vi "Check_EnFlo_Tunnel_Cond.vi"(2 "Averaging time (mins)":dbl=5.0, 3 "Traverse line":T1 {"Carrier_2 Q (l/min)" format="%#.2f"; "Row Duration (mins)" format="%#.1f"; "Row No" min=0; "Trace Gas Concentration (%)" min=0.0 format="%#_4f"; "Carrier_1 Q (l/min)" format="%#.4f"; "Start X" format="%#.2f"; "Start Y" format="%#.2f"; "Start Z" format="%#.2f"; "End X" format="%#.2f"; "End Y" format="%#.2f"; "End Z" format="%#.2f"; "Tunnel Speed" format="%#.2f"; "Averaging time (mins)" min=0.0 format="%#.2f"}) -> (0 "Status Cluster":T4, 1 "Heaters On?":bool)   [LabVIEW 2021]
uses:
  Anemometry/Anemometry Sub Vis/Gen Trav/Status_Cluster.ctl
  Anemometry/Anemometry Sub Vis/Gen Trav/Multi_Run_Status.ctl
  Anemometry/Anemometry Sub Vis/Gen Trav/Traverse_cluster.ctl
  Anemometry/Anemometry Sub Vis/Gen Trav/Spacing.ctl
  Anemometry/Anemometry Sub Vis/Controls/Multi_run_mode.ctl
  Anemometry/Anemometry Sub Vis/Controls/In_Range.ctl
  Anemometry/Anemometry Sub Vis/Controls/User_Specific_mode.ctl
  Anemometry/Anemometry Sub Vis/Globals/Meas_global.vi
  Anemometry/Anemometry Sub Vis/Globals/EnFlo_Tunnel_Global.vi
  Anemometry/Anemometry Sub Vis/Globals/Trav_pos_global.vi
panel:
  # "X           Y          Z"
  # "Start"
  # "End"
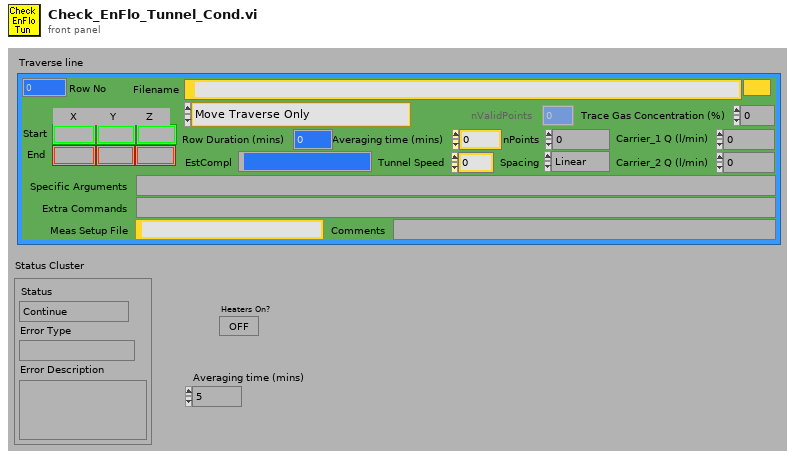
[diagram p1: front panel]
types:
  T1 = typedef "Traverse_cluster.ctl" = cluster{"Start X":sgl, "Start Y":sgl, "Start Z":sgl, "End X":sgl, "End Y":sgl, "End Z":sgl, "nPoints":i32, "Spacing":T2, "Filename":path, "Tunnel Speed":dbl, "Averaging time (mins)":dbl, "Extra Commands":string, "Carrier_1 Q (l/min)":dbl, "Carrier_2 Q (l/min)":dbl, "Trace Gas Concentration (%)":dbl, "Specific Arguments":string, "Comments":string, "Row No":i32, "Row Type Selector":T3, "EstCompl":string, "Row Duration (mins)":dbl, "nValidPoints":i32, "Meas Setup File":string}
  T2 = typedef "Spacing.ctl" = enum16{"Linear", "Log", "Gauss", "Specified", "N/A"}
  T3 = typedef "Multi_run_mode.ctl" = enum16{"Move Traverse Only", "Set Tunnel Speed Only", "Set Source Only", "Set Measurement Conditions", "Single Measurement", "Vertical Profile", "Lateral Profile", "Longitudinal Profile", "Multi-Axis Profile", "Explore Volume", "Auto Calibrate", "Meas Fast FID Bkgnd", "Check Beam Power", "Scanning Valve Measurement", "Run VI Named:", "Set ADAM Ch", "Wait (minutes)", "Send Message", "Synchronize With:", "Fall Back to this Row", "Turn Off Row Repeating", "Traverse 3D Volume", "Blank Row", "Jump to Fall Back Row"}
  T4 = typedef "Status_Cluster.ctl" = cluster{"Status":T5, "Error Type":string, "Error Description":string}
  T5 = typedef "Multi_Run_Status.ctl" = enum16{"Continue", "Continue with Error", "Jump to Next Point", "Jump to Next Row", "Jump To Fall Back", "Terminate Run"}
  T6 = typedef "In_Range.ctl" = enum16{"%", "±", "% & ±"}
  T7 = typedef "User_Specific_mode.ctl" = enum16{"Check VI only", "Run VI"}
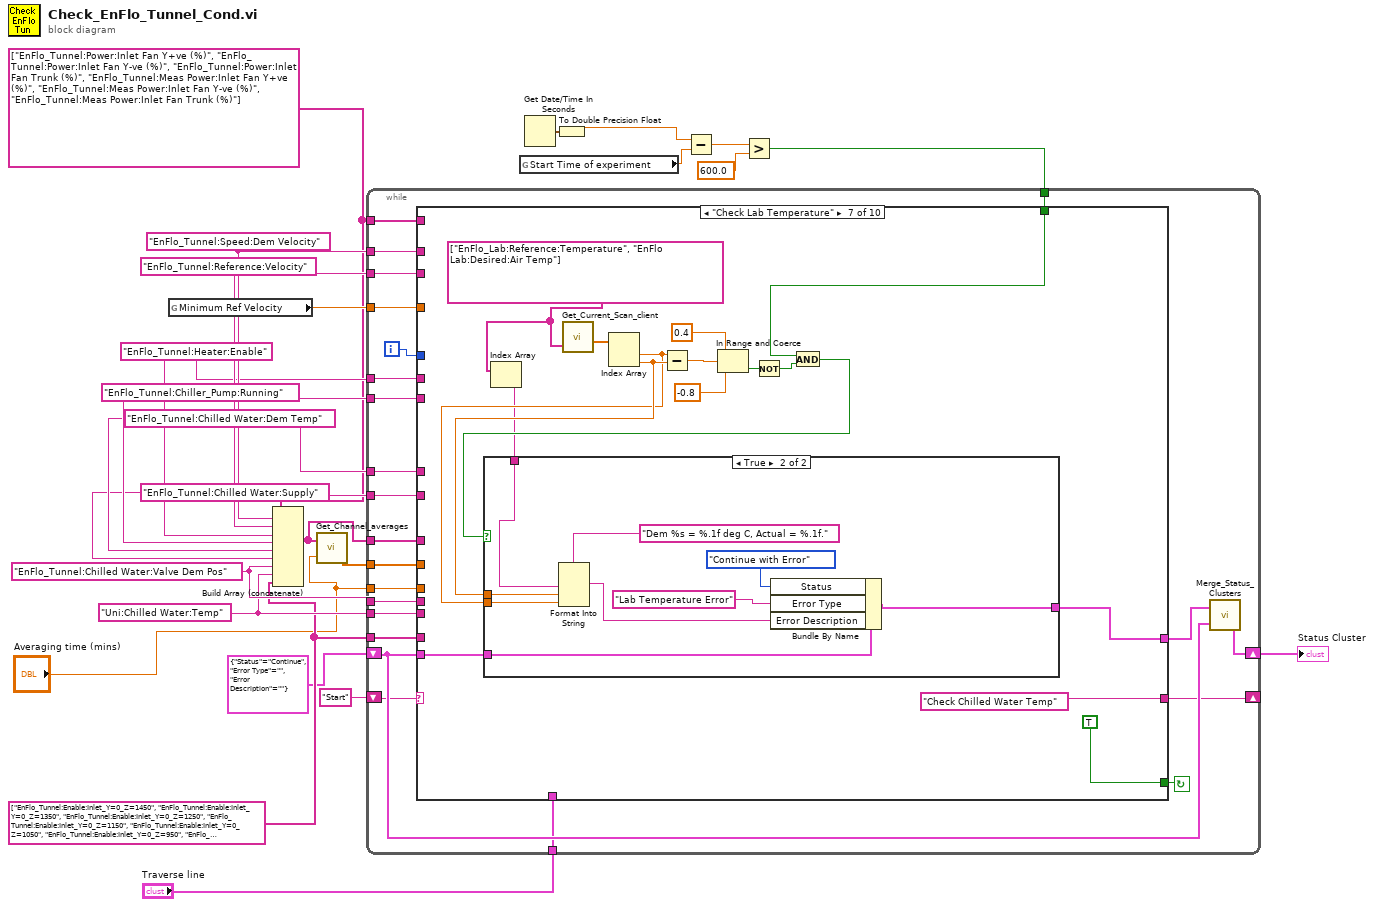
[diagram p0: block diagram]
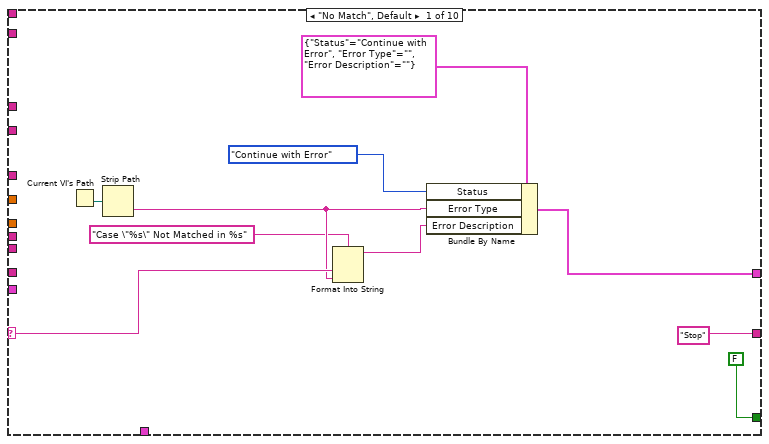
[diagram p2: hidden frame]
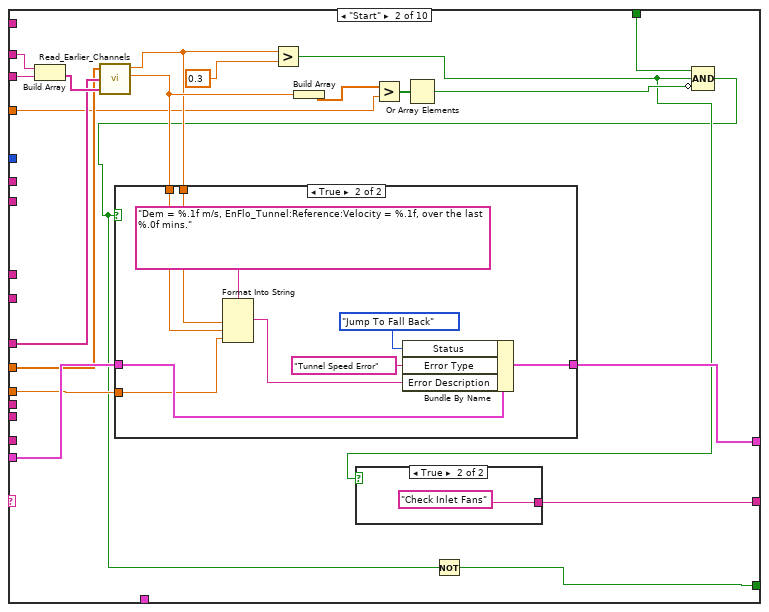
[diagram p3: hidden frame]
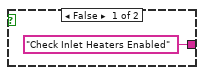
[diagram p4: hidden frame]
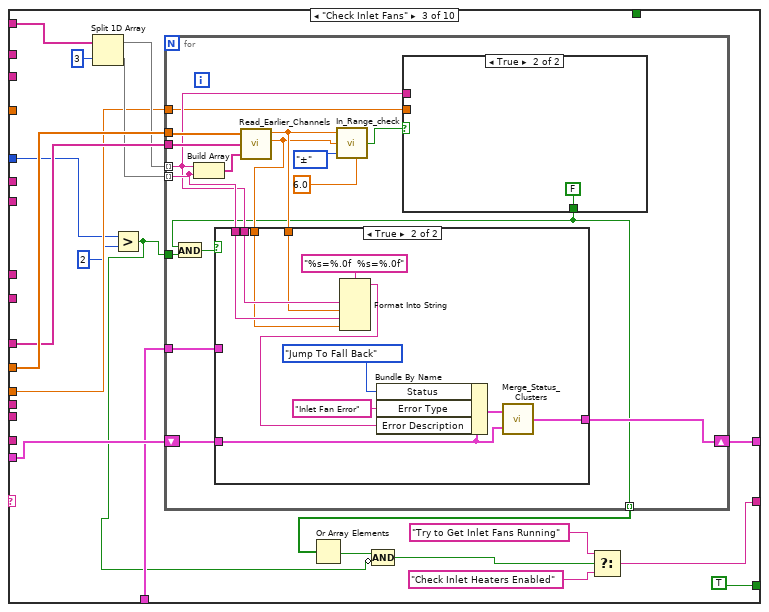
[diagram p6: hidden frame]
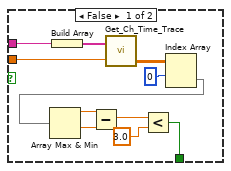
[diagram p7: hidden frame]
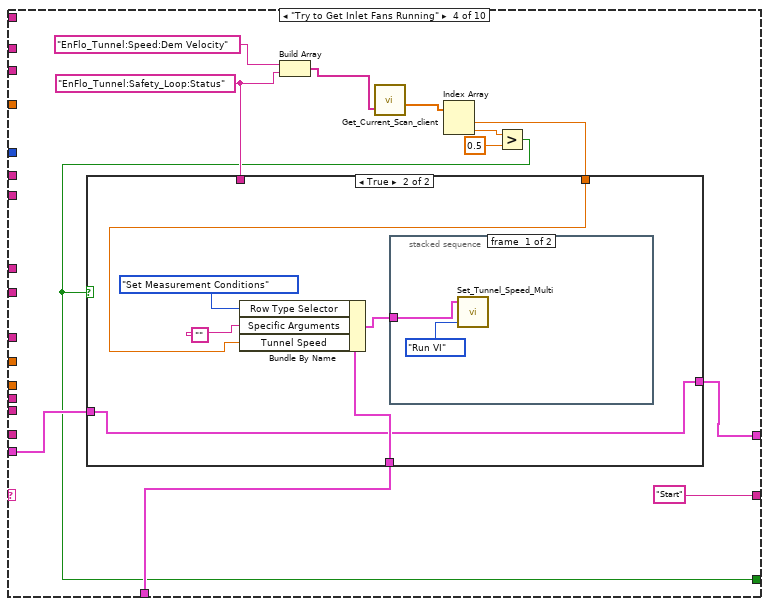
[diagram p9: hidden frame]
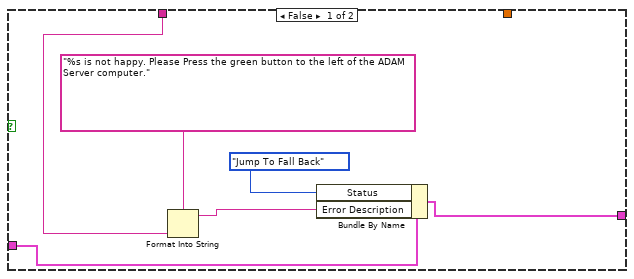
[diagram p10: hidden frame]
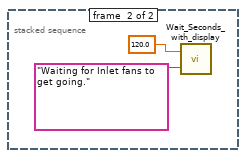
[diagram p11: hidden frame]
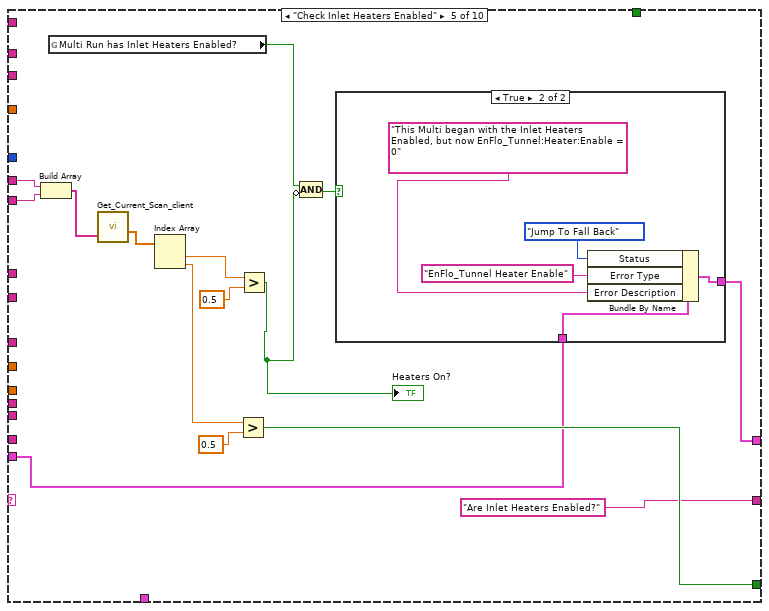
[diagram p12: hidden frame]
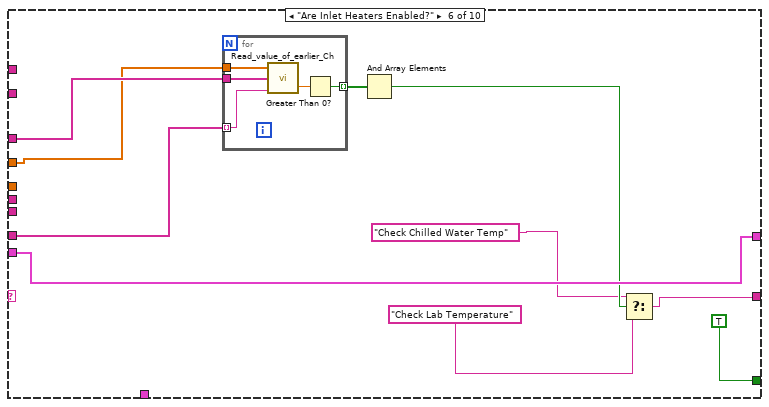
[diagram p14: hidden frame]
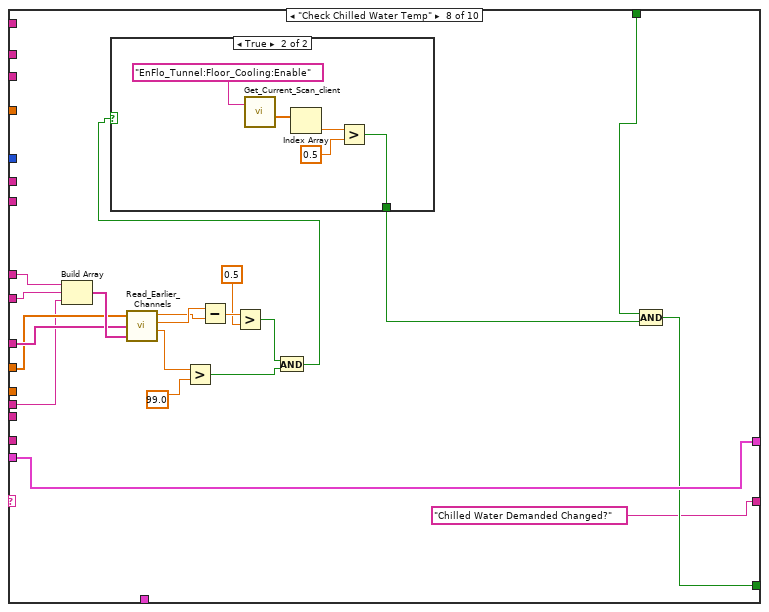
[diagram p16: hidden frame]
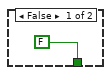
[diagram p17: hidden frame]
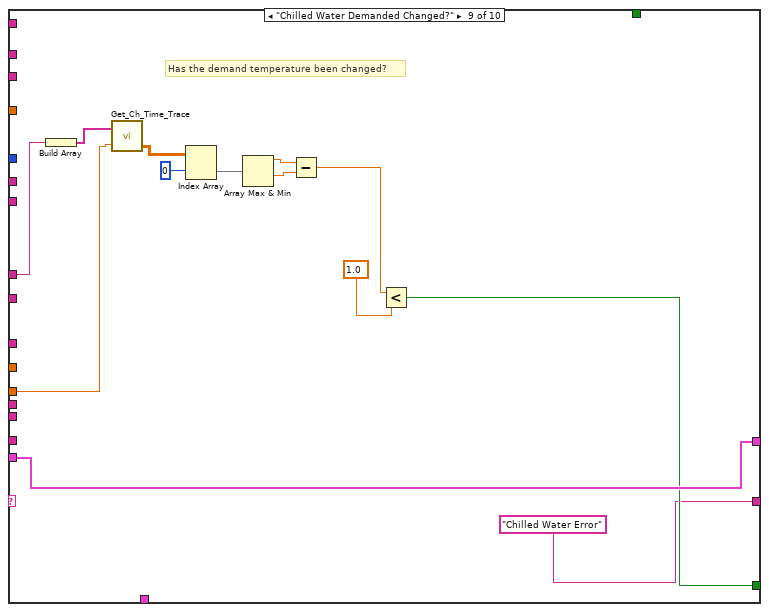
[diagram p18: hidden frame]
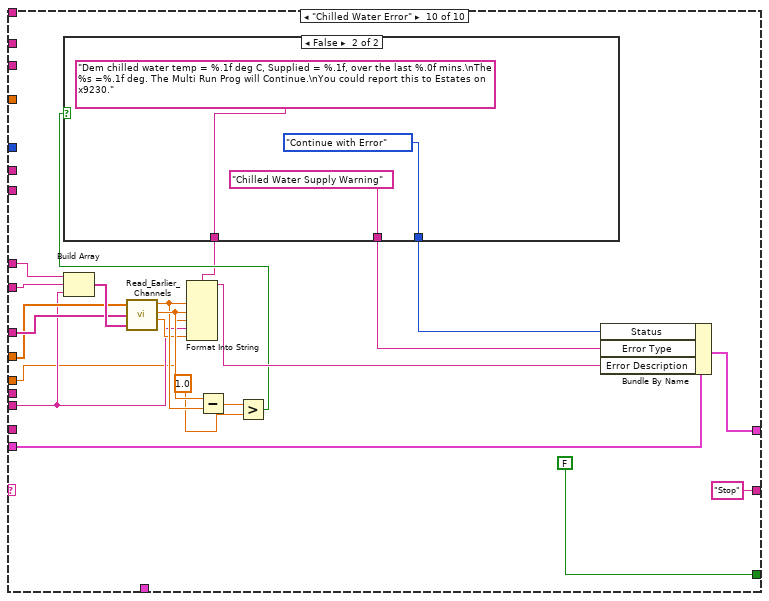
[diagram p19: hidden frame]
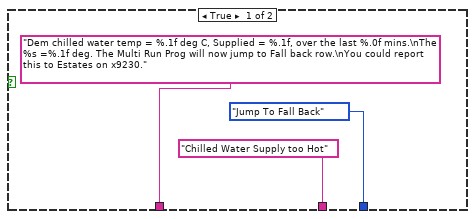
[diagram p20: hidden frame]
diagram:
  w6 = string[] ["EnFlo_Tunnel:Power:Inlet Fan Y+ve (%)", "EnFlo_Tunnel:Power:Inlet Fan Y-ve (%)", "EnFlo_Tunnel:Power:Inlet Fan Trunk (%)", "EnFlo_Tunnel:Meas Power:Inlet Fan Y+ve (%)", "EnFlo_Tunnel:Meas Power:Inlet Fan Y-ve (%)", "EnFlo_Tunnel:Meas Power:Inlet Fan Trunk (%)"] ("Sub set")
  w8 = string[] ["EnFlo_Tunnel:Enable:Inlet_Y=0_Z=1450", "EnFlo_Tunnel:Enable:Inlet_Y=0_Z=1350", "EnFlo_Tunnel:Enable:Inlet_Y=0_Z=1250", "EnFlo_Tunnel:Enable:Inlet_Y=0_Z=1150", "EnFlo_Tunnel:Enable:Inlet_Y=0_Z=1050", "EnFlo_Tunnel:Enable:Inlet_Y=0_Z=950", "EnFlo_Tunnel:Enable:Inlet_Y=0_Z=850", "EnFlo_Tunnel:Enable:Inlet_Y=0_Z=750", "EnFlo_Tunnel:Enable:Inlet_Y=0_Z=650", "EnFlo_Tunnel:Enable:Inlet_Y=0_Z=550", "EnFlo_Tunnel:Enable:Inlet_Y=0_Z=450", "EnFlo_Tunnel:Enable:Inlet_Y=0_Z=350", "EnFlo_Tunnel:Enable:Inlet_Y=0_Z=250", "EnFlo_Tunnel:Enable:Inlet_Y=0_Z=150", "EnFlo_Tunnel:Enable:Inlet_Y=0_Z=50"] ("Sub set")
  w9 = "Uni:Chilled Water:Temp"
  w10 = "EnFlo_Tunnel:Chilled Water:Valve Dem Pos"
  w17 = "EnFlo_Tunnel:Chilled Water:Supply"
  w18 = "EnFlo_Tunnel:Chilled Water:Dem Temp"
  w19 = "EnFlo_Tunnel:Chiller_Pump:Running"
  w21 = "EnFlo_Tunnel:Heater:Enable"
  w23 = "EnFlo_Tunnel:Speed:Dem Velocity"
  w22 = "EnFlo_Tunnel:Reference:Velocity"
  n1 = global read "EnFlo_Tunnel_Global.vi" "Minimum Ref Velocity"() -> (w7:dbl)
  n2 = Build Array (concatenate)(w6, w23, w22, w21, w19, w18, w17, w10, w9, w8) -> (w20:string[])
  n3 = call "Get_Channel_averages.vi"("Desired Ch Names"=w20, "Averaging time (mins)"="Averaging time (mins)") -> ("number"=w24:dbl[])  [unwired: 1 in, 2 out]
  n4 = global read "Meas_global.vi" "Start Time of experiment"() -> (w14:dbl)
  n5 = Get Date/Time In Seconds() -> (seconds since 1Jan1904=w11:timestamp)
  n6 = To Double Precision Float(number=w11) -> (double precision float=w13:dbl)
  n7 = Subtract(x=w13, y=w14) -> (x-y=w15:dbl)
  n8 = Greater?(x=w15, y=600.0) -> (0:w12:bool)
  n9 = while {
    tunnel: w12 -> [w33]
    tunnel: w17 -> [w34]
    tunnel: w18 -> [w35]
    tunnel: w19 -> [w36]
    shift-left: "Start" -> [w38]
    shift-right: [w37] -> _
    tunnel: w21 -> [w42]
    tunnel: w22 -> [w43]
    tunnel: w23 -> [w44]
    tunnel: w20 -> [w45]
    tunnel: w24 -> [w46]
    shift-left: T4 {"Status"=enum."Continue", "Error Type"="", "Error Description"=""} ("Status Cluster In") -> [w40]
    shift-right: [w39] -> w4
    tunnel: "Averaging time (mins)" -> [w32]
    tunnel: w10 -> [w31]
    tunnel: w9 -> [w30]
    tunnel: w8 -> [w29]
    tunnel: w7 -> [w28]
    tunnel: w6 -> [w27]
    tunnel: "Traverse line" -> [w26]
    i -> [w25]
    stop <- w47 continue-if-true
    n10 = case shown="\"Check Lab Temperature\"" w38 {
      selector: w38 -> [w51 _ _ _ _ _ _ _ _ _]
      tunnel: [FALSE w58 TRUE w152 w192 TRUE TRUE w253 w276 FALSE] -> w47
      tunnel: w46 -> [_ w71 w107 _ _ w205 _ w257 _ w298]
      tunnel: w45 -> [_ w72 w106 _ _ w206 _ w258 _ w299]
      tunnel: w44 -> [_ w75 _ _ _ _ _ _ _ _]
      tunnel: w43 -> [_ w74 _ _ _ _ _ _ _ _]
      tunnel: w40 -> [_ w77 w103 w157 w187 w209 w228 w260 w279 w291]
      tunnel: [w54 w76 w102 w151 w186 w209 w227 w260 w279 w290] -> w41
      tunnel: w42 -> [_ _ _ _ w183 _ _ _ _ _]
      tunnel: ["Stop" w61 w92 "Start" "Are Inlet Heaters Enabled?" w207 "Check Chilled Water Temp" "Chilled Water Demanded Changed?" "Chilled Water Error" "Stop"] -> w37
      tunnel: w36 -> [_ _ _ _ w182 _ _ _ _ _]
      tunnel: w35 -> [_ _ _ _ _ _ _ w256 w275 w296]
      tunnel: w34 -> [_ _ _ _ _ _ _ w255 _ w297]
      tunnel: w33 -> [_ w65 _ _ _ _ w224 w254 _ _]
      tunnel: w32 -> [_ w60 w100 _ _ _ _ _ w273 w281]
      tunnel: w31 -> [_ _ _ _ _ _ _ w251 _ _]
      tunnel: w30 -> [_ _ _ _ _ _ _ _ _ w282]
      tunnel: w29 -> [_ _ _ _ _ w204 _ _ _ _]
      tunnel: w28 -> [_ w64 _ _ _ _ _ _ _ _]
      tunnel: w27 -> [_ _ w109 _ _ _ _ _ _ _]
      tunnel: w26 -> [_ _ w99 w162 _ _ _ _ _ _]
      tunnel: w25 -> [_ _ w98 _ _ _ _ _ _ _]
      frame "No Match", Default {
        n11 = Current VI's Path() -> (path=w52:path)
        n12 = Strip Path(path=w52) -> (name=w50:string)  [unwired: 1 out]
        n13 = Format Into String(format string="Case \"%s\" Not Matched in %s", w51, w50) -> (resulting string=w48:string)  [unwired: 2 in, 1 out]
        n14 = Bundle By Name(cluster=T4 {"Status"=enum."Continue with Error", "Error Type"="", "Error Description"=""} ("Status Cluster In"), "Status"=Multi_Run_Status."Continue with Error", "Error Type"=w50, "Error Description"=w48) -> (w54:T4)
      }
      frame "Start" {
        n15 = Build Array(w75, w74) -> (w73:string[])
        n16 = call "Read_Earlier_Channels.vi"("Present scan array"=w71, "Ch names"=w72, "Desired Channels"=w73) -> ("Index 0"=w69:dbl, "Index 1"=w70:dbl)  [unwired: 4 out]
        n17 = Greater?(x=w69, y=0.3) -> (0:w62:bool)
        n18 = Build Array(w70) -> (w67:dbl[])
        n19 = case shown="True" w62 {
          tunnel: ["Check Inlet Heaters Enabled" "Check Inlet Fans"] -> w61
          frame False {
          }
          frame True {
          }
        }
        n20 = Greater?(x=w67, y=w64) -> (0:w66:bool[])
        n21 = Or Array Elements(Boolean array=w66) -> (logical OR=w63:bool)
        n22 = Compound Arithmetic op=AND(w65, w62, invert w63) -> (w59:bool)
        n23 = case shown="True" w59 {
          tunnel: [w80 w88] -> w76
          tunnel: w77 -> [w80 w89]
          tunnel: w69 -> [_ w83]
          tunnel: w70 -> [_ w82]
          tunnel: w60 -> [_ w81]
          frame False {
          }
          frame True {
            n24 = Format Into String(format string="Dem = %.1f m/s, EnFlo_Tunnel:Reference:Velocity = %.1f, over the last %.0f mins." ("Format String"), w83, w82, w81) -> (resulting string=w84:string)  [unwired: 2 in, 1 out]
            n25 = Bundle By Name(cluster=w89, "Status"=Multi_Run_Status."Jump To Fall Back", "Error Type"="Tunnel Speed Error" ("Bundle Element"), "Error Description"=w84) -> (w88:T4)
          }
        }
        n26 = Not(x=w59) -> (.not. x?=w58:bool)
      }
      frame "Check Inlet Fans" {
        n27 = Split 1D Array(array=w109, index=3) -> (first subarray=w105:string[], second subarray=w104:string[])
        n28 = Greater?(x=w98, y=2) -> (0:w94:bool)
        n29 = for {
          tunnel: w107 -> [w126]
          tunnel: w106 -> [w125]
          tunnel: w105 -> [w115] mode=indexing
          tunnel: w104 -> [w120] mode=indexing
          shift-right: [w117] -> w102
          shift-left: w103 -> [w118]
          tunnel: w100 -> [w114]
          tunnel: w99 -> [w113]
          tunnel: w94 -> [w111]
          tunnel: [w110] -> w96 mode=indexing
          n30 = Build Array(w115, w120) -> (w122:string[])
          n31 = call "Read_Earlier_Channels.vi"("Present scan array"=w126, "Ch names"=w125, "Desired Channels"=w122) -> ("Index 0"=w121:dbl, "Index 1"=w119:dbl)  [unwired: 4 out]
          n32 = call "In_Range_check.vi"("±"=6.0, "Mode"=In_Range."±", "Value"=w119, "Setpoint"=w121) -> ("In Range"=w116:bool)  [unwired: 3 in]
          n33 = case shown="True" w116 {
            tunnel: w115 -> [w137 _]
            tunnel: w114 -> [w128 _]
            tunnel: [w127 FALSE] -> w110
            frame False {
              n34 = Build Array(w137) -> (w136:string[])
              n35 = call "Get_Ch_Time_Trace.vi"("Desired Ch Names"=w136, "History Length (mins)"=w128) -> ("Output array"=w135:dbl[][])  [unwired: 2 out]
              n36 = Index Array(array=w135, index (row)=0) -> (element=w133:dbl[])  [unwired: 1 in]
              n37 = Array Max & Min(array=w133) -> (max value=w132:dbl, min value=w131:dbl)  [unwired: 2 out]
              n38 = Subtract(x=w132, y=w131) -> (x-y=w130:dbl)
              n39 = Less?(x=w130, y=3.0) -> (x < y?=w127:bool)
            }
            frame True {
            }
          }
          n40 = And(x=w110, y=w111) -> (x .and. y?=w112:bool)
          n41 = case shown="True" w112 {
            tunnel: w115 -> [_ w150]
            tunnel: w121 -> [_ w149]
            tunnel: w120 -> [_ w148]
            tunnel: w119 -> [_ w147]
            tunnel: w118 -> [w139 w141]
            tunnel: [w139 w140] -> w117
            tunnel: w113 -> [_ _]
            frame False {
            }
            frame True {
              n42 = Format Into String(format string="%s=%.0f  %s=%.0f", w150, w149, w148, w147) -> (resulting string=w143:string)  [unwired: 2 in, 1 out]
              n43 = Bundle By Name(cluster=w141, "Status"=Multi_Run_Status."Jump To Fall Back", "Error Type"="Inlet Fan Error" ("Bundle Element"), "Error Description"=w143) -> (w142:T4)
              n44 = call "Merge_Status_Clusters.vi"("Status Cluster 2"=w141, "Status Cluster 1"=w142) -> ("Status Cluster Out"=w140:T4)
            }
          }
        }
        n45 = Or Array Elements(Boolean array=w96) -> (logical OR=w95:bool)
        n46 = Compound Arithmetic op=AND(w95, invert w94) -> (w93:bool)
        n47 = Select(t="Try to Get Inlet Fans Running", s=w93, f="Check Inlet Heaters Enabled") -> (s? t:f=w92:string)
      }
      frame "Try to Get Inlet Fans Running" {
        w154 = "EnFlo_Tunnel:Safety_Loop:Status"
        n48 = Build Array("EnFlo_Tunnel:Speed:Dem Velocity", w154) -> (w155:string[])
        n49 = call "Get_Current_Scan_client.vi"("multipleChannels"=w155) -> ("Numerical Values"=w161:dbl[])  [unwired: 1 in, 3 out]
        n50 = Index Array(array=w161) -> (element #1=w160:dbl, element #2=w159:dbl)  [unwired: 2 in]
        n51 = Greater?(x=w159, y=0.5) -> (0:w152:bool)
        n52 = case shown="True" w152 {
          tunnel: w162 -> [_ w174]
          tunnel: w160 -> [_ w170]
          tunnel: w157 -> [w165 w169]
          tunnel: w154 -> [w168 _]
          tunnel: [w163 w169] -> w151
          frame False {
            n53 = Format Into String(format string="%s is not happy. Please Press the green button to the left of the ADAM Server computer.", w168) -> (resulting string=w167:string)  [unwired: 2 in, 1 out]
            n54 = Bundle By Name(cluster=w165, "Status"=Multi_Run_Status."Jump To Fall Back", "Error Description"=w167) -> (w163:T4)
          }
          frame True {
            n55 = Bundle By Name(cluster=w174, "Row Type Selector"=Multi_run_mode."Set Measurement Conditions", "Specific Arguments"="", "Tunnel Speed"=w170) -> (w171:T1)
            n56 = stacked-sequence {
              tunnel: w171 -> [w176 _]
              frame #0 {
                n57 = call "Set_Tunnel_Speed_Multi.vi"("Simulate/Run"=User_Specific_mode."Run VI", "Traverse line"=w176) -> ()  [unwired: 4 out]
              }
              frame #1 {
                n58 = call "Wait_Seconds_with_display.vi"("Message"="Waiting for Inlet fans to get going.", "Seconds to wait"=120.0) -> ()  [unwired: 1 in, 1 out]
              }
            }
          }
        }
      }
      frame "Check Inlet Heaters Enabled" {
        n59 = Build Array(w183, w182) -> (w185:string[])
        n60 = global read "Trav_pos_global.vi" "Multi Run has Inlet Heaters Enabled?"() -> (w190:bool)
        n61 = call "Get_Current_Scan_client.vi"("multipleChannels"=w185) -> ("Numerical Values"=w184:dbl[])  [unwired: 1 in, 3 out]
        n62 = Index Array(array=w184) -> (element #1=w181:dbl, element #2=w180:dbl)  [unwired: 2 in]
        n63 = Greater?(x=w180, y=0.5) -> (0:w192:bool)
        n64 = Greater?(x=w181, y=0.5) -> (0:w189:bool)
        "Heaters On?" <- w189
        n65 = Compound Arithmetic op=AND(w190, invert w189) -> (w188:bool)
        n66 = case shown="True" w188 {
          tunnel: w187 -> [w194 w197]
          tunnel: [w194 w196] -> w186
          frame False {
          }
          frame True {
            n67 = Bundle By Name(cluster=w197, "Status"=Multi_Run_Status."Jump To Fall Back", "Error Type"="EnFlo_Tunnel Heater Enable" ("Bundle Element"), "Error Description"="This Multi began with the Inlet Heaters Enabled, but now EnFlo_Tunnel:Heater:Enable = 0") -> (w196:T4)
          }
        }
      }
      frame "Are Inlet Heaters Enabled?" {
        n68 = for {
          tunnel: w205 -> [w214]
          tunnel: w206 -> [w213]
          tunnel: w204 -> [w212] mode=indexing
          tunnel: [w210] -> w203 mode=indexing
          n69 = call "Read_value_of_earlier_Ch.vi"("Desired Ch to Read"=w212, "Ch names"=w213, "Present scan array"=w214) -> ("Value"=w211:dbl)  [unwired: 1 in, 1 out]
          n70 = Greater Than 0?(x=w211) -> (x > 0?=w210:bool)
        }
        n71 = And Array Elements(Boolean array=w203) -> (logical AND=w202:bool)
        n72 = Select(t="Check Chilled Water Temp", s=w202, f="Check Lab Temperature") -> (s? t:f=w207:string)
      }
      frame "Check Lab Temperature" {
        w222 = string[] ["EnFlo_Lab:Reference:Temperature", "EnFlo Lab:Desired:Air Temp"] ("appended array")
        n73 = Index Array(array=w222) -> (element=w221:string)  [unwired: 1 in]
        n74 = call "Get_Current_Scan_client.vi"("multipleChannels"=w222) -> ("Numerical Values"=w230:dbl[])  [unwired: 1 in, 3 out]
        n75 = Index Array(array=w230) -> (element #1=w225:dbl, element #2=w226:dbl)  [unwired: 2 in]
        n76 = Subtract(x=w225, y=w226) -> (x-y=w219:dbl)
        n77 = In Range and Coerce(upper limit=0.4 ("abs(x)"), x=w219, lower limit=-0.8 ("abs(x)")) -> (In Range?=w216:bool)  [unwired: 1 out]
        n78 = Not(x=w216) -> (.not. x?=w215:bool)
        n79 = And(x=w224, y=w215) -> (x .and. y?=w223:bool)
        n80 = case shown="True" w223 {
          tunnel: w228 -> [w231 w237]
          tunnel: [w231 w236] -> w227
          tunnel: w226 -> [_ w235]
          tunnel: w225 -> [_ w234]
          tunnel: w221 -> [_ w232]
          frame False {
          }
          frame True {
            n81 = Format Into String(format string="Dem %s = %.1f deg C, Actual = %.1f." ("Format String"), w232, w235, w234) -> (resulting string=w238:string)  [unwired: 2 in, 1 out]
            n82 = Bundle By Name(cluster=w237, "Status"=Multi_Run_Status."Continue with Error", "Error Type"="Lab Temperature Error" ("Bundle Element"), "Error Description"=w238) -> (w236:T4)
          }
        }
      }
      frame "Check Chilled Water Temp" {
        n83 = Build Array(w256, w255, w251) -> (w259:string[])
        n84 = call "Read_Earlier_Channels.vi"("Present scan array"=w257, "Ch names"=w258, "Desired Channels"=w259) -> ("Index 0"=w249:dbl, "Index 1"=w250:dbl, "Index 2"=w246:dbl)  [unwired: 3 out]
        n85 = Greater?(x=w246, y=99.0) -> (0:w244:bool)
        n86 = Subtract(x=w250, y=w249) -> (x-y=w248:dbl)
        n87 = Greater?(x=w248, y=0.5) -> (0:w243:bool)
        n88 = And(x=w243, y=w244) -> (x .and. y?=w242:bool)
        n89 = case shown="True" w242 {
          tunnel: [FALSE w263] -> w252
          frame False {
          }
          frame True {
            n90 = call "Get_Current_Scan_client.vi"("singleChannel"="EnFlo_Tunnel:Floor_Cooling:Enable") -> ("Numerical Values"=w266:dbl[])  [unwired: 1 in, 3 out]
            n91 = Index Array(array=w266) -> (element=w265:dbl)  [unwired: 1 in]
            n92 = Greater?(x=w265, y=0.5) -> (0:w263:bool)
          }
        }
        n93 = Compound Arithmetic op=AND(w254, w252) -> (w253:bool)
      }
      frame "Chilled Water Demanded Changed?" {
        # "Has the demand temperature been changed?"
        n94 = Build Array(w275) -> (w274:string[])
        n95 = call "Get_Ch_Time_Trace.vi"("Desired Ch Names"=w274, "History Length (mins)"=w273) -> ("Output array"=w272:dbl[][])  [unwired: 2 out]
        n96 = Index Array(array=w272, index (row)=0 ("Index")) -> (element=w271:dbl[])  [unwired: 1 in]
        n97 = Array Max & Min(array=w271) -> (max value=w270:dbl, min value=w269:dbl)  [unwired: 2 out]
        n98 = Subtract(x=w270, y=w269) -> (x-y=w268:dbl)
        n99 = Less?(x=w268, y=1.0) -> (x < y?=w276:bool)
      }
      frame "Chilled Water Error" {
        n100 = Build Array(w296, w297, w282) -> (w300:string[])
        n101 = call "Read_Earlier_Channels.vi"("Present scan array"=w298, "Ch names"=w299, "Desired Channels"=w300) -> ("Index 0"=w288:dbl, "Index 1"=w289:dbl, "Index 2"=w284:dbl)  [unwired: 3 out]
        n102 = Subtract(x=w289, y=w288) -> (x-y=w287:dbl)
        n103 = Greater?(x=w287, y=1.0) -> (0:w285:bool)
        n104 = case shown="False" w285 {
          tunnel: [Multi_Run_Status."Jump To Fall Back" ("Status") Multi_Run_Status."Continue with Error" ("Status")] -> w294
          tunnel: ["Chilled Water Supply too Hot" ("Bundle Element") "Chilled Water Supply Warning" ("Bundle Element")] -> w293
          tunnel: ["Dem chilled water temp = %.1f deg C, Supplied = %.1f, over the last %.0f mins.\nThe %s =%.1f deg. The Multi Run Prog will now jump to Fall back row.\nYou could report this to Estates on x9230." ("Format String") "Dem chilled water temp = %.1f deg C, Supplied = %.1f, over the last %.0f mins.\nThe %s =%.1f deg. The Multi Run Prog will Continue.\nYou could report this to Estates on x9230." ("Format String")] -> w283
          frame True {
          }
          frame False {
          }
        }
        n105 = Format Into String(format string=w283, w288, w289, w281, w282, w284) -> (resulting string=w292:string)  [unwired: 2 in, 1 out]
        n106 = Bundle By Name(cluster=w291, "Status"=w294, "Error Type"=w293, "Error Description"=w292) -> (w290:T4)
      }
    }
    n107 = call "Merge_Status_Clusters.vi"("Status Cluster 2"=w40, "Status Cluster 1"=w41) -> ("Status Cluster Out"=w39:T4)
  }
  "Status Cluster" <- w4
